vi "Settings Panel.vi"(8 "error in (no error)":errorcluster, 10 "MainUI":refnum<queue>, 11 "SettingQueue":refnum<queue>) -> (0 "error out":errorcluster)   [LabVIEW 2019, in "Settings.lvlib"]
doc: "Dialog for selecting user specified settings."
uses:
  Settings.lvlib
  MainController/Cluster - MainControllerMessage.ctl
  MainController/Enum - MainState.ctl
  CTL_MessageCluster.ctl
  CTL_SettingsMessage.ctl
  Cluster - Settings.ctl
  MainController/Cluster - HardwareConfiguration.ctl
  MainController/Cluster - TestSettings.ctl
  <vilib>/Utility/error.llb/DialogType.ctl
  <vilib>/Utility/xml.llb/Write to XML File(string).vi
  MainController/MainController.lvlib
panel:
  in  "Save":bool
  in  "Output Data Base Path":path
  in  "AutoIncrement":bool
  # "Auto Mode"
  # "Logging"
  # "About"
  # "This text should contain a brief description about this application."
  # "Version: 1.0.0.0"
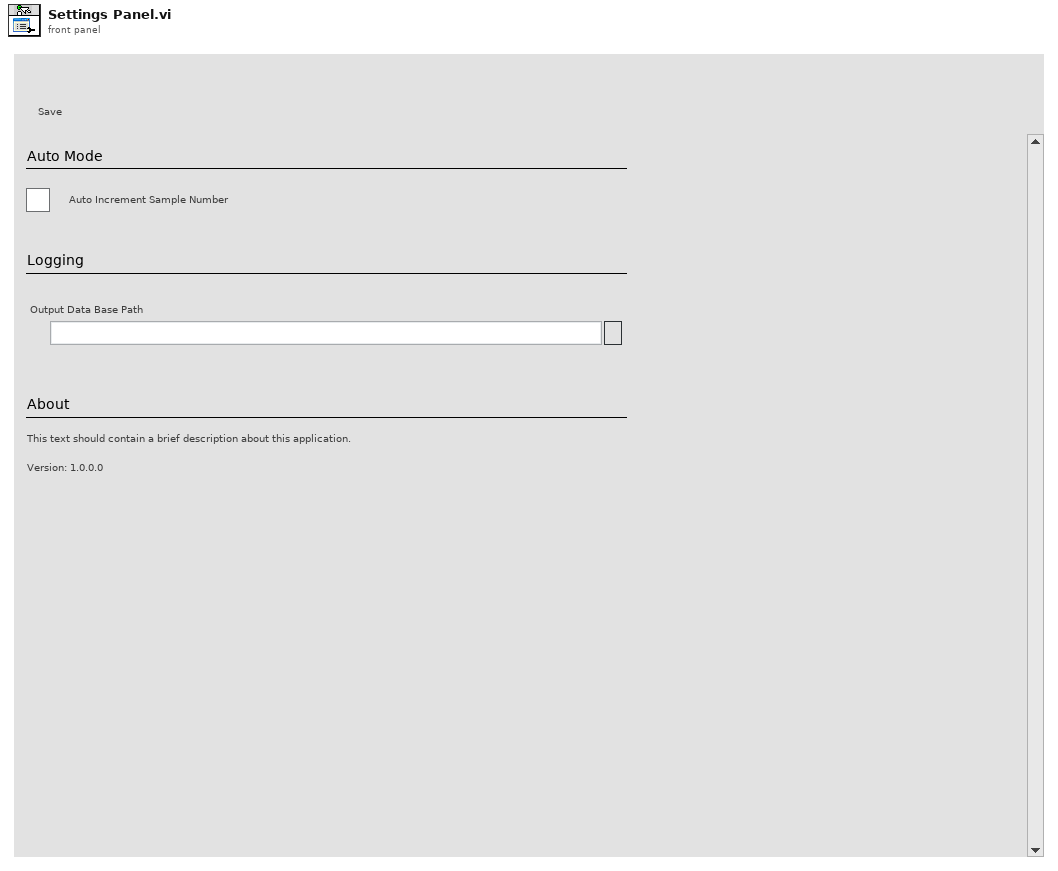
[diagram p1: front panel]
types:
  T1 = typedef "Settings.lvlib/CTL_SettingsMessage.ctl" = enum16{"Inititalize", "Idle", "LoadSettings", "SaveSettings", "Exit"}
  T2 = typedef "Settings.lvlib/Cluster - Settings.ctl" = cluster{"Hardware Configuration":T3, "TestSettings":T4}
  T3 = typedef "MainController.lvlib/Cluster - HardwareConfiguration.ctl" = cluster{"Mark10COM":refnum<visa-resource-name>, "IsConnected":bool}
  T4 = typedef "MainController.lvlib/Cluster - TestSettings.ctl" = cluster{"Sample":u32, "Applicator Prefix":string, "Winding Distance":dbl, "Winding Speed":dbl, "Dwell Time":dbl, "Auto Increment Sample":bool, "Output Data Path":path, "File Base Path":path}
  T5 = typedef "Settings.lvlib/CTL_MessageCluster.ctl" = cluster{"Message":T1, "Data":variant}
  T6 = typedef "MainController.lvlib/Enum - MainState.ctl" = enum16{"Initialize", "InitUIRefs", "LaunchSettings", "LaunchAutoMode", "LaunchManualMode", "LaunchTestReport", "ConnectHardware", "DisconnectHardware", "HiliteNavItems", "StartAutoMode", "PauseAutoMode", "StopAutoMode", "ShowFlyout", "HideFlyout", "BroadcastSettings", "PickupTestSettings", "BroadcastHW", "AutoTestDone", "DAQStatus", "UpdateCommandBar", "Error", "RecieveError", "Exit"}
  T7 = typedef "DialogType.ctl" = u16
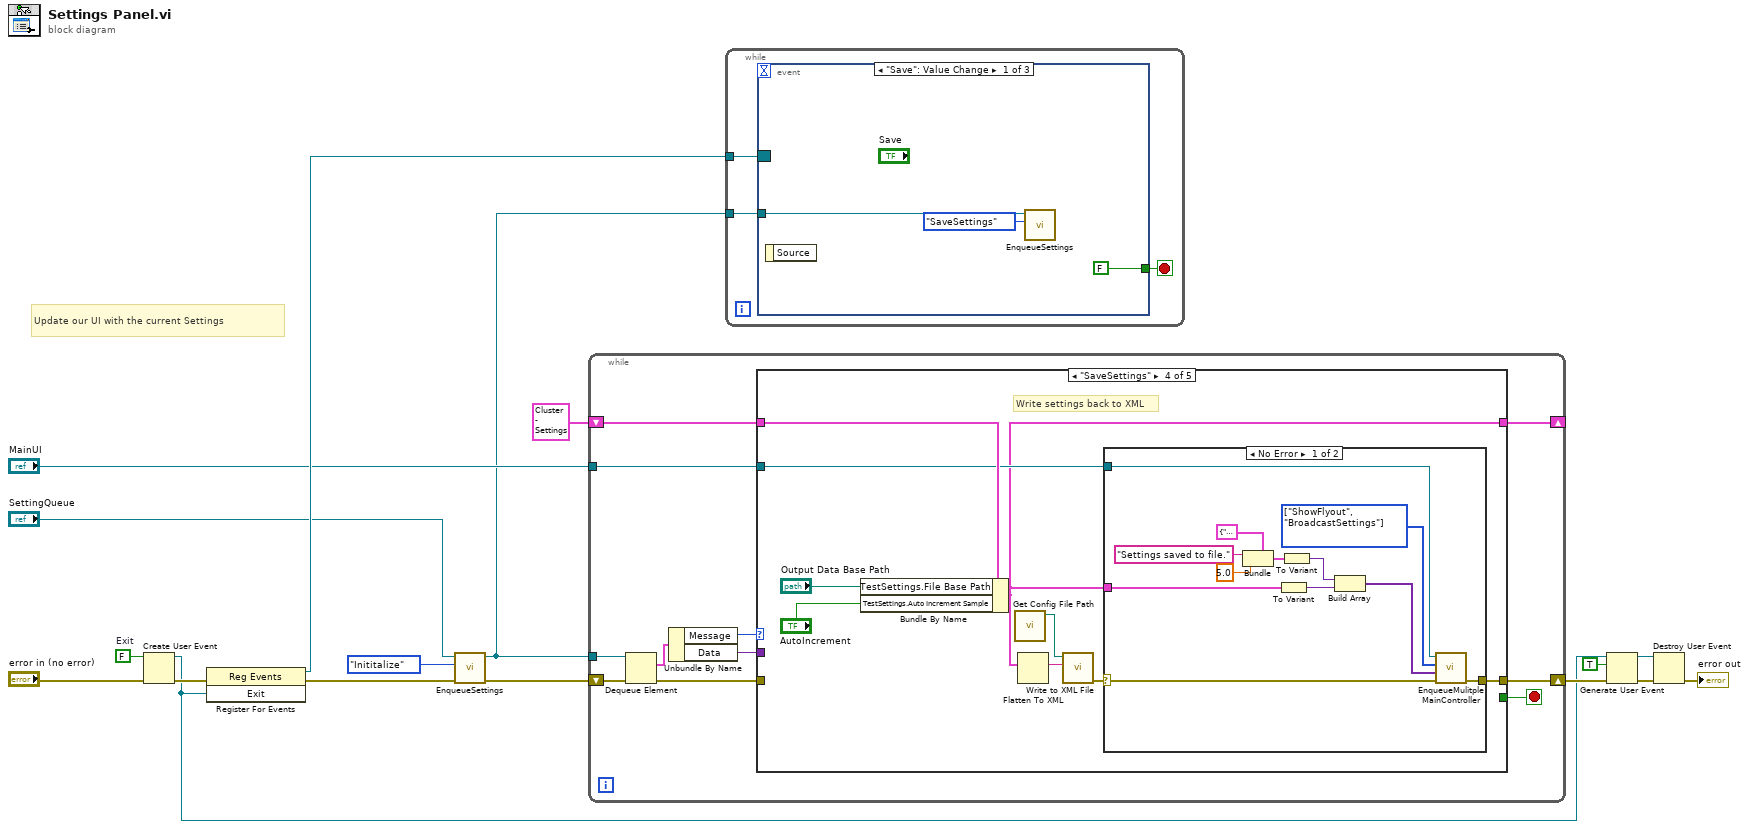
[diagram p0: block diagram]
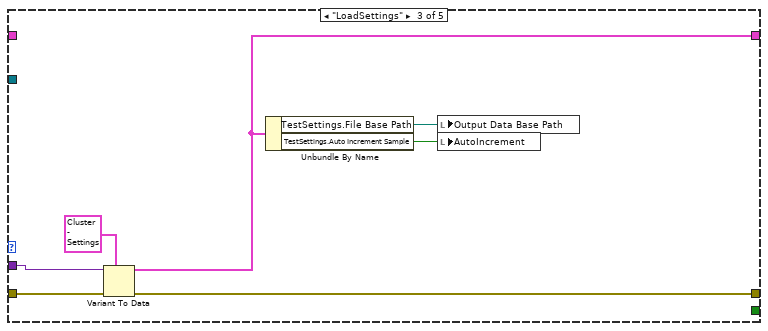
[diagram p4: hidden frame]
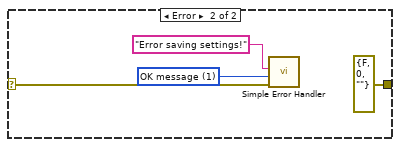
[diagram p5: hidden frame]
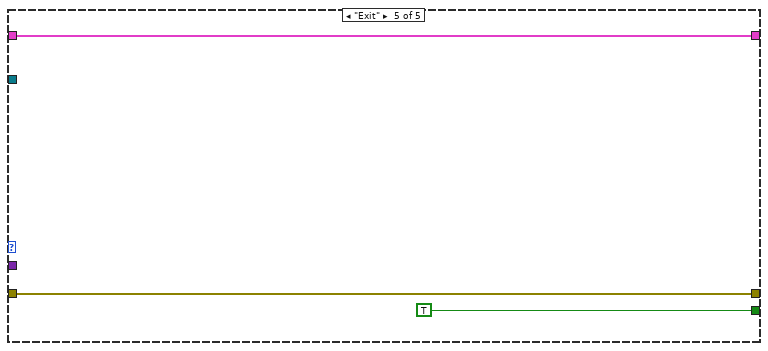
[diagram p6: hidden frame]
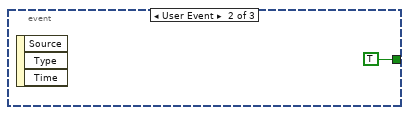
[diagram p7: hidden frame]
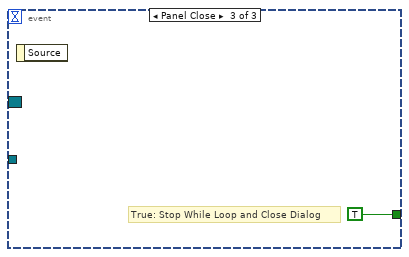
[diagram p8: hidden frame]
diagram:
  w14 = FALSE  # Exit
  # "Update our UI with the current Settings"
  n1 = Create User Event(user event datatype=w14, error in="error in (no error)") -> (user event=w10:refnum<user-event>, error out=w15:errorcluster)
  n2 = register-events(error in=w15, w10) -> (reference out=w13:refnum<event-registration>, error out=w5:errorcluster)  [unwired: 1 in]
  n3 = call "EnqueueSettings.vi"("error in (no error)"=w5, "Message"=CTL_SettingsMessage."Inititalize", "SettingsQueue"="SettingQueue") -> ("error out"=w2:errorcluster, "queue out"=w1:refnum<queue>)  [unwired: 7 in]
  n4 = while {
    tunnel: w1 -> [w27]
    shift-right: [w23] -> w16
    shift-left: w2 -> [w28]
    shift-right: [w20] -> _
    shift-left: T2 {"Hardware Configuration"={"Mark10COM"="", "IsConnected"=FALSE}, "TestSettings"={"Sample"=0, "Applicator Prefix"="", "Winding Distance"=0.0, "Winding Speed"=0.0, "Dwell Time"=0.0, "Auto Increment Sample"=FALSE, "Output Data Path"=path "C:/Users/adammi/Google Drive/LabVIEW/PatchRotationFixture/Reports", "File Base Path"=path ""}} ("Settings in") -> [w21]
    tunnel: "MainUI" -> [w18]
    stop <- w19 stop-if-true
    n5 = Dequeue Element(queue=w27, error in (no error)=w28) -> (element=w26:T5, error out=w22:errorcluster)  [unwired: 1 in, 2 out]
    n6 = Unbundle By Name(w26) -> ("Message"=w25:T1, "Data"=w24:variant)
    n7 = case shown="\"SaveSettings\"" w25 {
      tunnel: w24 -> [_ _ w35 _ _]
      tunnel: [w30 w32 w36 w43 w67] -> w23
      tunnel: w22 -> [w30 w32 w39 _ w67]
      tunnel: w21 -> [w29 w31 _ w45 w66]
      tunnel: [w29 w31 w33 w42 w66] -> w20
      tunnel: [_ _ _ _ TRUE] -> w19
      tunnel: w18 -> [_ _ _ w44 _]
      frame "Inititalize", Default {
      }
      frame "Idle" {
      }
      frame "LoadSettings" {
        n8 = Variant To Data(error in=w39, type=T2 {"Hardware Configuration"={"Mark10COM"="", "IsConnected"=FALSE}, "TestSettings"={"Sample"=0, "Applicator Prefix"="", "Winding Distance"=0.0, "Winding Speed"=0.0, "Dwell Time"=0.0, "Auto Increment Sample"=FALSE, "Output Data Path"=path "C:/Users/adammi/Google Drive/LabVIEW/PatchRotationFixture/Reports", "File Base Path"=path ""}} ("Settings in"), Variant=w35) -> (data=w33:T2, error out=w36:errorcluster)
        n9 = Unbundle By Name(w33) -> ("TestSettings.File Base Path"=w37:path, "TestSettings.Auto Increment Sample"=w38:bool)
        n10 = local write "Output Data Base Path"(w37) -> ()
        n11 = local write "AutoIncrement"(w38) -> ()
      }
      frame "SaveSettings" {
        # "Write settings back to XML"
        n12 = Bundle By Name(cluster=w45, "TestSettings.File Base Path"="Output Data Base Path", "TestSettings.Auto Increment Sample"="AutoIncrement") -> (w42:T2)
        n13 = call "Get Config File Path.vi"() -> ("XML File Path"=w47:path)  [unwired: 10 in, 1 out]
        n14 = Flatten To XML(anything=w42) -> (xml string=w48:string)
        n15 = call-poly <vilib>:"Write to XML File.vi"("XML Input"=w48, "XML File Path"=w47) -> ("error out"=w46:errorcluster)  [unwired: 7 in, 2 out]
        n16 = case shown="No Error" w46 {
          selector: w46 -> [w60 w63]
          tunnel: w44 -> [w59 _]
          tunnel: [w56 errorcluster {"status"=FALSE, "code"=0, "source"=""} ("error out")] -> w43
          tunnel: w42 -> [w55 _]
          frame No Error {
            w58 = T6[] [enum."ShowFlyout", enum."BroadcastSettings"] items=["Initialize", "InitUIRefs", "LaunchSettings", "LaunchAutoMode", "LaunchManualMode", "LaunchTestReport", "ConnectHardware", "DisconnectHardware", "HiliteNavItems", "StartAutoMode", "PauseAutoMode", "StopAutoMode", "ShowFlyout", "HideFlyout", "BroadcastSettings", "PickupTestSettings", "BroadcastHW", "AutoTestDone", "DAQStatus", "UpdateCommandBar", "Error", "RecieveError", "Exit"] ("Messages")
            n17 = Bundle(cluster=cluster{"Message":string, "Timeout":dbl} {"Message"="", "Timeout"=0.0}, "Message"="Settings saved to file.", "Timeout"=5.0) -> (w49:cluster{"Message":string, "Timeout":dbl})
            n18 = To Variant(anything=w55) -> (Variant=w53:variant)
            n19 = To Variant(anything=w49) -> (Variant=w54:variant)
            n20 = Build Array(w54, w53) -> (w57:variant[])
            n21 = call "EnqueueMulitpleMainController.vi"("error in (no error)"=w60, "Data"=w57, "Messages"=w58, "MainQueue"=w59) -> ("error out"=w56:errorcluster)  [unwired: 5 in, 2 out]
          }
          frame Error {
            w62 = T7 1 items=["no dialog", "OK message", "continue or stop message", "OK message + warnings", "continue/stop + warnings"] ("type of dialog (OK msg:1)")
            n22 = call <vilib>:"Simple Error Handler.vi"("error source (\" \")"="Error saving settings!", "type of dialog (OK msg:1)"=w62, "error in (no error)"=w63) -> ()  [unwired: 2 in, 5 out]
          }
        }
      }
      frame "Exit" {
      }
    }
  }
  n23 = while {
    tunnel: w13 -> [w69]
    tunnel: w1 -> [w68]
    stop <- w70 stop-if-true
    n24 = event shown="[0] \"Save\": Value Change" {
      selector: w69 -> [_ _ _]
      dyn-events: _ -> [_ _ _]
      timeout: _ -> [_ _ _]
      tunnel: [FALSE TRUE TRUE] -> w70
      tunnel: w68 -> [w72 _ _]
      event "Save": Value Change {
        n25 = event-data() -> ()  [unwired: 1 in, 1 out]
        n26 = call "EnqueueSettings.vi"("Message"=CTL_SettingsMessage."SaveSettings", "SettingsQueue"=w72) -> ()  [unwired: 8 in, 2 out]
      }
      event User Event {
        n27 = event-data() -> ()  [unwired: 1 in, 3 out]
      }
      event Panel Close {
        # "True: Stop While Loop and Close Dialog"
        n28 = event-data() -> ()  [unwired: 1 in, 1 out]
      }
    }
  }
  n29 = Generate User Event(user event=w10, event data cluster=TRUE ("event data"), error in=w16) -> (user event out=w9:refnum<user-event>, error out=w11:errorcluster)  [unwired: 1 in]
  n30 = Destroy User Event(user event=w9, error in=w11) -> (error out=→"error out":errorcluster)
